vi "buildTestScenario.vi"(0 "TestScenarioFactory in":refnum<class "TestScenarioFactory.lvclass">, 5 "Log":refnum<class "ITestLog.lvclass">, 7 "Test Scenario":T1, 11 "error in (no error)":errorcluster) -> (4 "TestScenarioFactory out":refnum<class "TestScenarioFactory.lvclass">, 6 "ITestScenario.lvclass":refnum<class "ITestScenario.lvclass">, 15 "error out":errorcluster)   [LabVIEW 2015, in "TestScenarioFactory.lvclass"]
uses:
  TestScenarioFactory.lvclass
  Typedefs/TestScenarioTypes.ctl
  TestScenario/ITestScenario/ITestScenario.lvclass
  TestLog/ITestLog/ITestLog.lvclass
  TestScenario/Not Implemented Test/NotImplementedTest.lvclass
  TestScenario/Constant Analog Output Voltage Test/Constant Analog Output Voltage Test.lvclass
  TestScenarioFactory.lvclass/TestScenarioFactory.ctl
  TestScenario/SSR_TTL Low Test/SSR_TTL Low Test.lvclass
  TestScenario/SSR_TTL High Test/SSR_TTL High Test.lvclass
  TestScenario/SM_CW Low Test/SM_CW Low Test.lvclass
  TestScenario/SM_CW High Test/SM_CW High Test.lvclass
  TestScenario/SM_CCW Low Test/SM_CCW Low Test.lvclass
  TestScenario/SM_CCW High Test/SM_CCW High Test.lvclass
  TestScenario/RS232-TXD Low Test/RS232-TXD Low Test.lvclass
  TestScenario/RS232-TXD High Test/RS232-TXD High Test.lvclass
  TestScenario/RS232-RTS Low Test/RS232-RTS Low Test.lvclass
  TestScenario/RS232-RTS High Test/RS232-RTS High Test.lvclass
  TestScenario/RS232-RXD Low Test/RS232-RXD Low Test.lvclass
  TestScenario/RS232-RXD High Test/RS232-RXD High Test.lvclass
  TestScenario/RS232-CTS low Test/RS232-CTS low Test.lvclass
  TestScenario/RS232-CTS High Test/RS232-CTS High Test.lvclass
  TestScenario/Modulated Analog Output Voltage Test/Modulated Analog Output Voltage Test.lvclass
  ConfigureILCStrategy/ConfigureILCROTStrategy/ConfigureILCROTStrategy.lvclass
  ConverterStrategy/ConvertROTRawToEngStrategy/ConvertROTRawToEngStrategy.lvclass
  ConfigureILCStrategy/ConfigureILCDAC1Strategy/ConfigureILCDAC1Strategy.lvclass
  ConverterStrategy/ConvertDACRawToEngStrategy/ConvertDACRawToEngStrategy.lvclass
  Typedefs/ILCBTTypedefs.lvlib
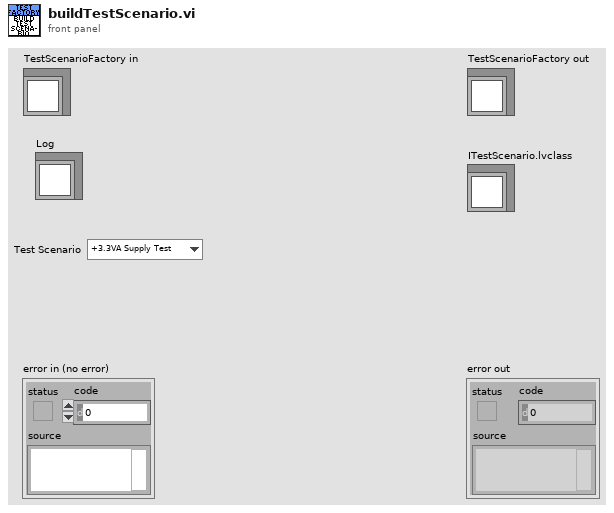
[diagram p1: front panel]
types:
  T1 = typedef "ILCBTTypedefs.lvlib/TestScenarioTypes.ctl" = enum16{"+3.3VA Supply Test", "+3.3VD Supply Test", "+5VA Supply Test", "+5VD Supply Test", "Unique ID Test", "TEDS Status Test", "LIMSW1_TTL Low Test", "LIMSW1_TTL High Test", "LIMSW2_TTL Low Test", "LIMSW2_TTL High Test", "Tachometer Test", "SSR_TTL Low Test", "SSR_TTL High Test", "SM_CW Low Test", "SM_CW High Test", "SM_CCW Low Test", "SM_CCW High Test", "SM_GPI Low Test", "SM_GPI High Test", "CW Motion Without Limit Test", "CW Motion With Limit Test", "CW Motion With Limit Interruption Test", "CW Motion on CCW Limit Test", "CCW Motion Without Limit Test", "CCW Motion With Limit Test", "CCW Motion With Limit Interruption Test", "CCW Motion on CW Limit Test", "RS232-TXD Low Test", "RS232-TXD High Test", "RS232-RTS Low Test", "RS232-RTS High Test", "RS232-RXD Low Test", "RS232-RXD High Test", "RS232-CTS Low Test", "RS232-CTS High Test", "Out_SS Low Test", "Out_SS High Test", "Out_SDI Low Test", "Out_SDI High Test", "Out_SCLK Low Test", "Out_SCLK High Test", "Reset Low Test", "Reset High Test", "1 Channel ADC Test", "3 Channel ADC Test", "5 Channel ADC Test", "Vref Test", "ROT Test", "DAC1 Test", "DAC2 Test", "DAC3 Test", "DAC4 Test", "BIAS Test", "EXC1 Test", "EXC2 Test", "EXC3 Test", "EXC4 Test"}
  T2 = typedef "ILCBTTypedefs.lvlib/ILC Digital Output Test.ctl" = cluster{"DAQ Channel to Read":refnum<k21>, "High Level Value to Test":T3, "High Level Value to Expect":T3, "Low Level Value to Test":T3, "Low Level Value to Expect":T3}
  T3 = typedef "ILCBTTypedefs.lvlib/Digital Signal Level.ctl" = enum16{"Low", "High"}
  T4 = typedef "ILCBTTypedefs.lvlib/MUX Settings.ctl" = cluster{"MUX_AO":T3, "MUX_A1":T3, "MUX_A0 DAQ Channel to Write":refnum<k21>, "MUX_A1 DAQ Channel to Write":refnum<k21>}
  T5 = typedef "ILCBTTypedefs.lvlib/Test Values.ctl" = cluster{"Start Value":dbl, "Stop Value":dbl, "Number of Steps":u16}
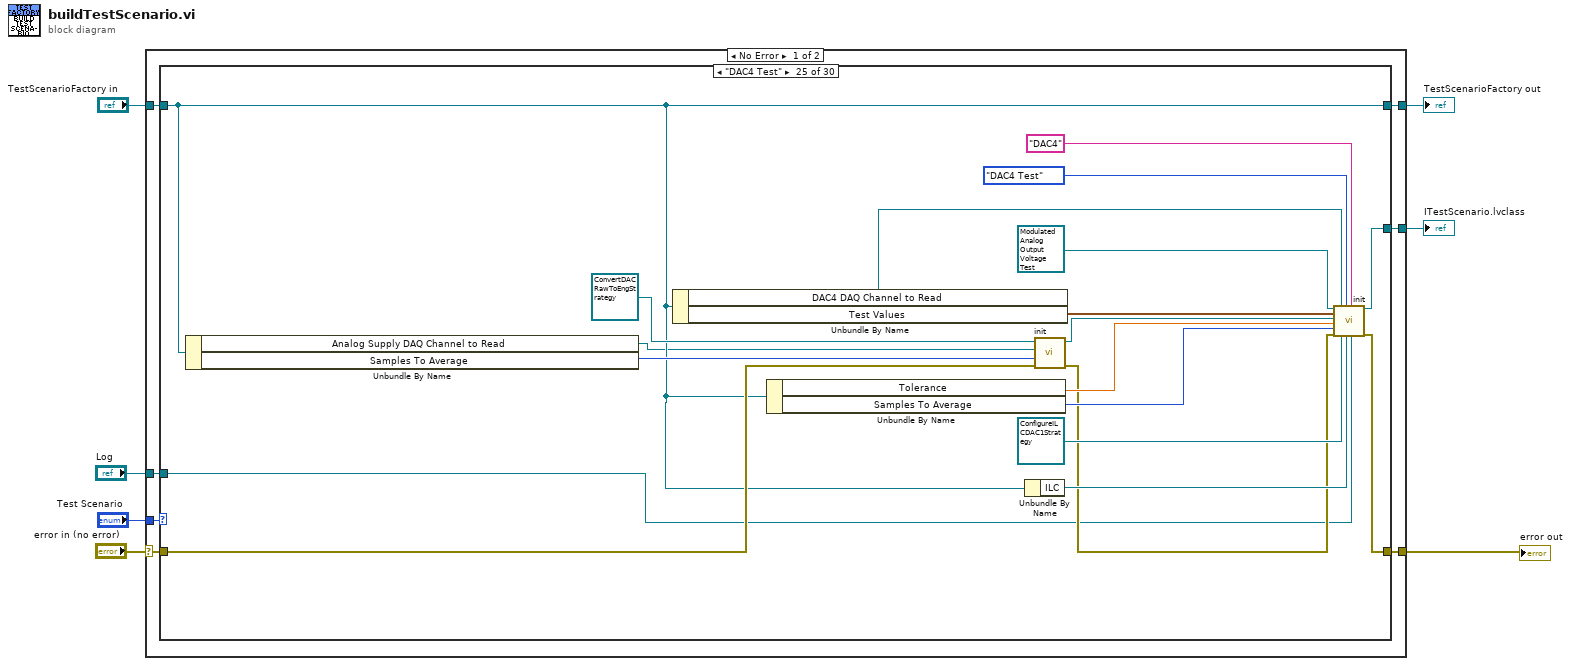
[diagram p0: block diagram]
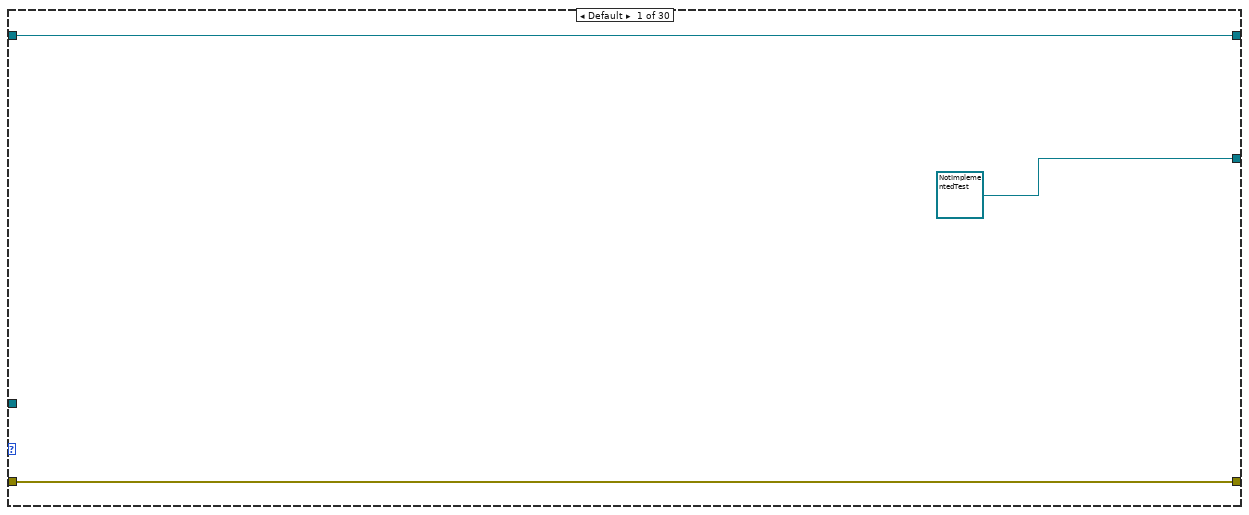
[diagram p2: hidden frame]
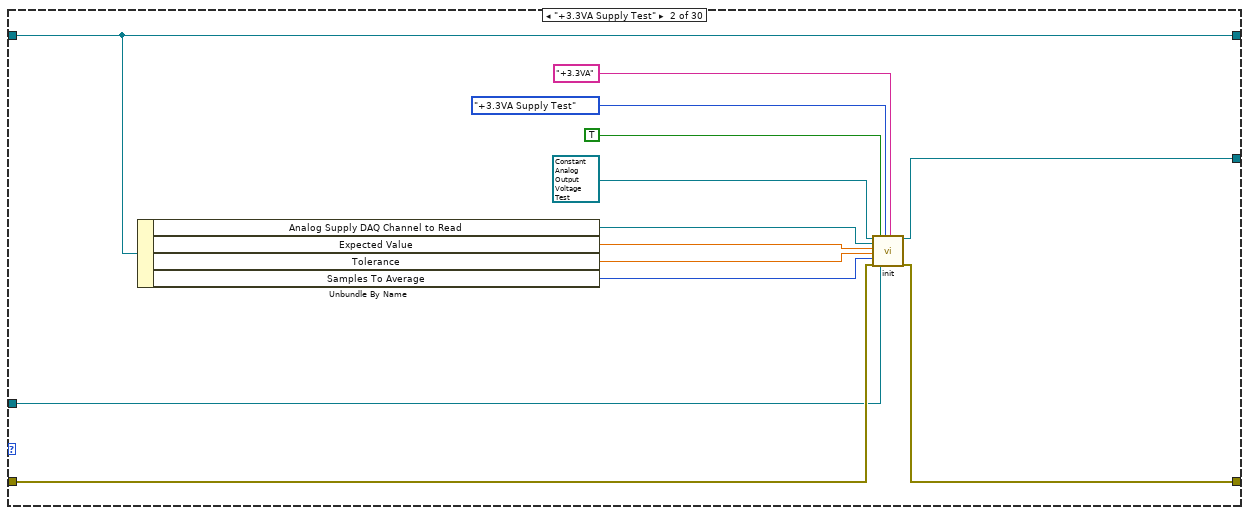
[diagram p3: hidden frame]
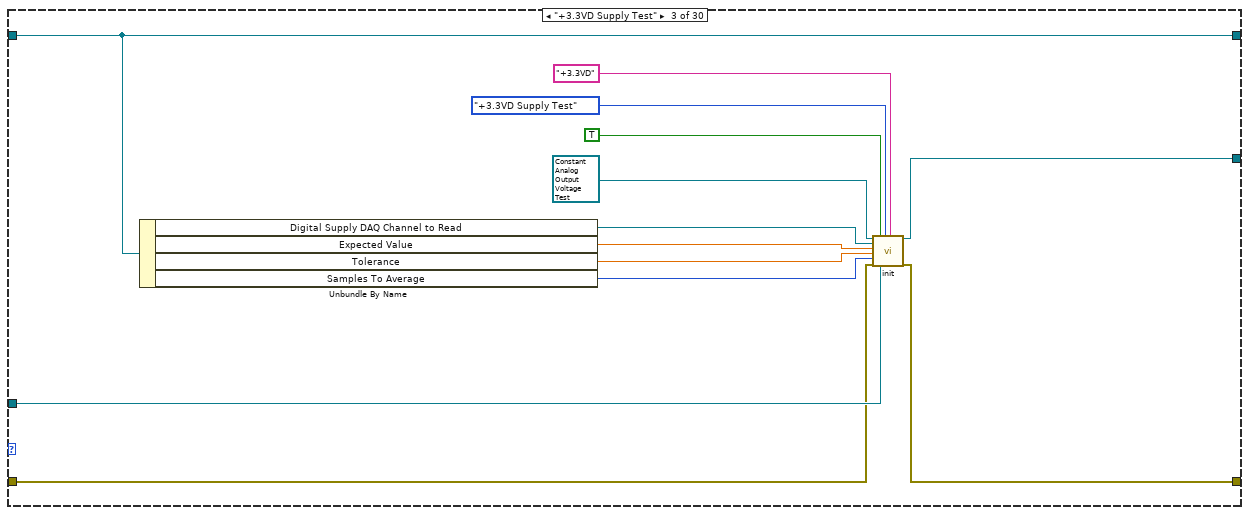
[diagram p4: hidden frame]
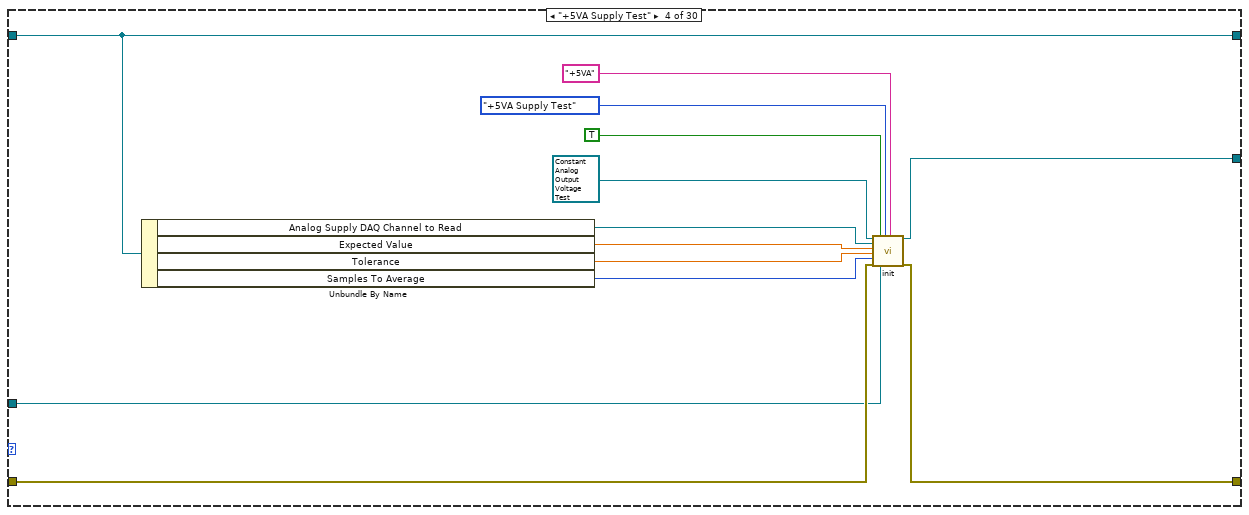
[diagram p5: hidden frame]
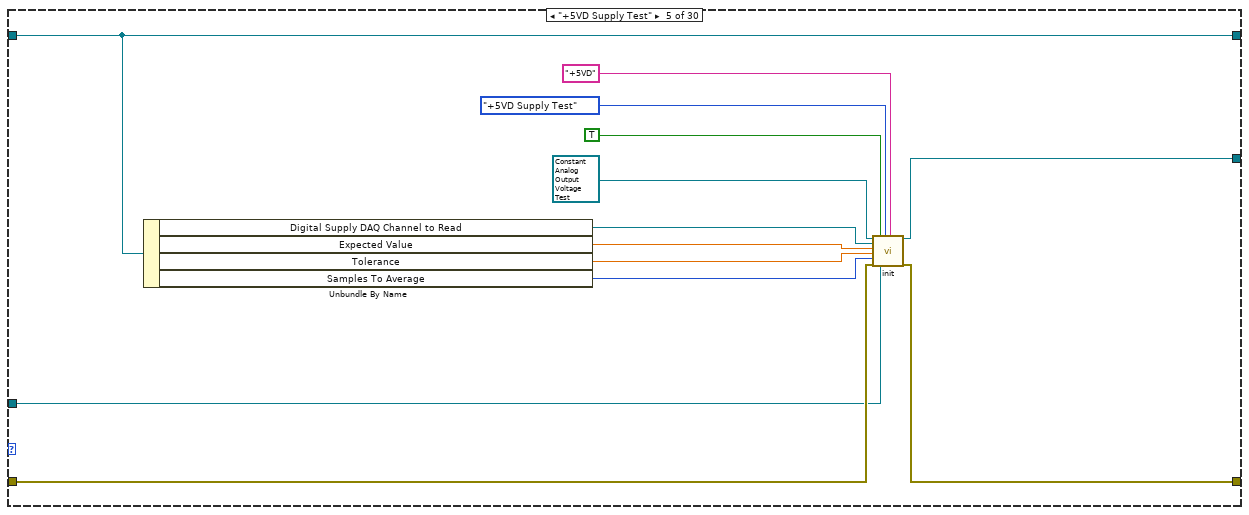
[diagram p6: hidden frame]
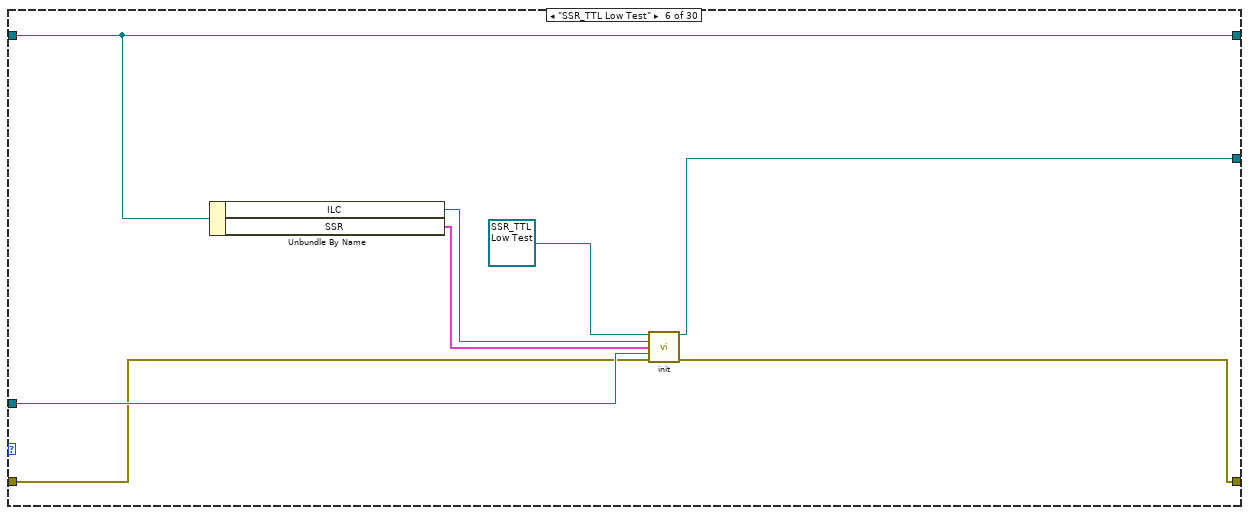
[diagram p7: hidden frame]
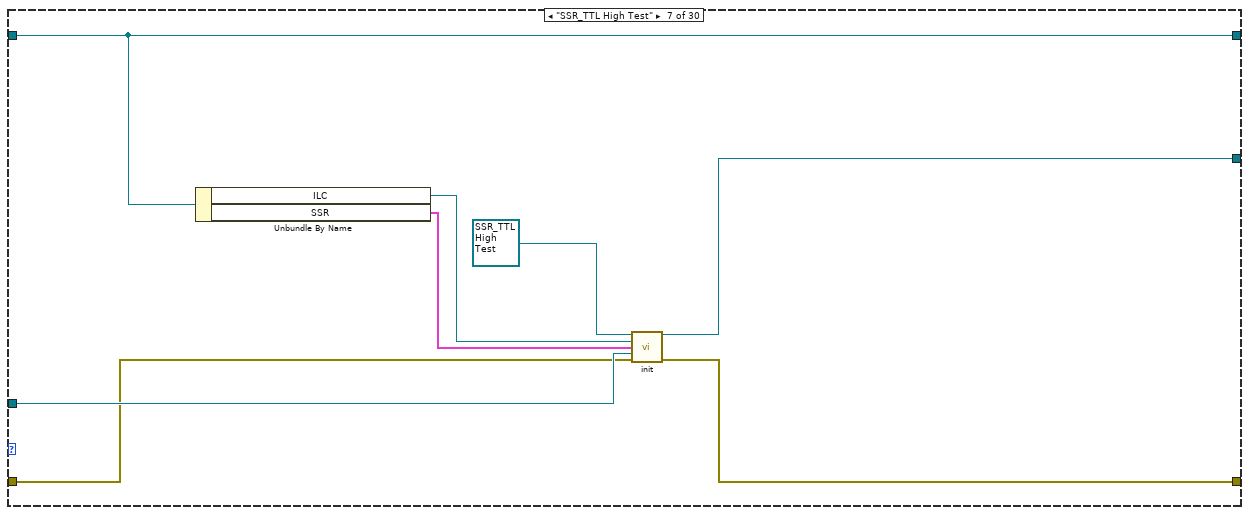
[diagram p8: hidden frame]
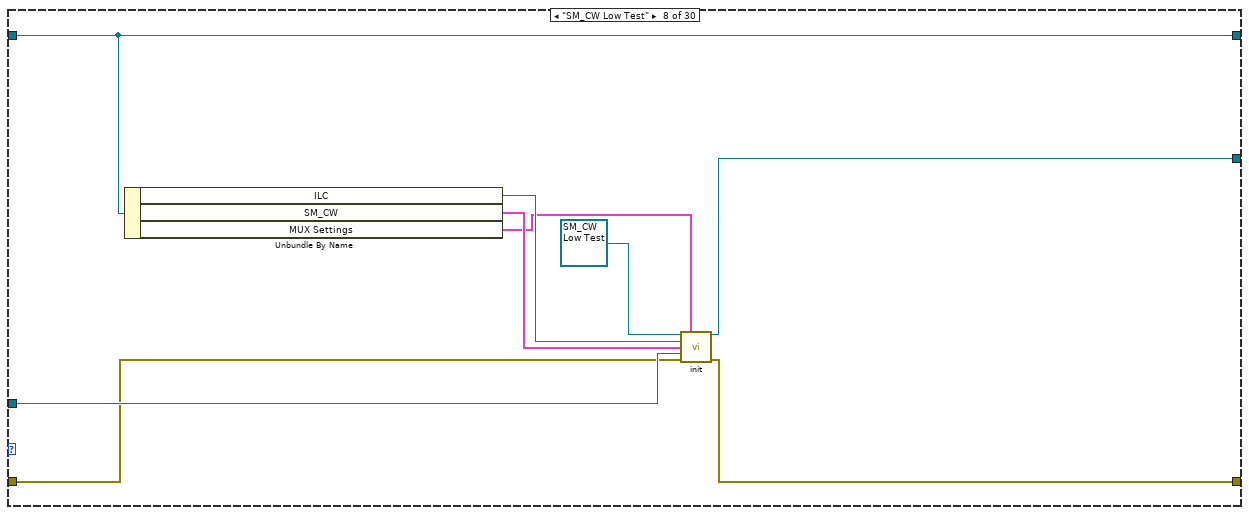
[diagram p9: hidden frame]
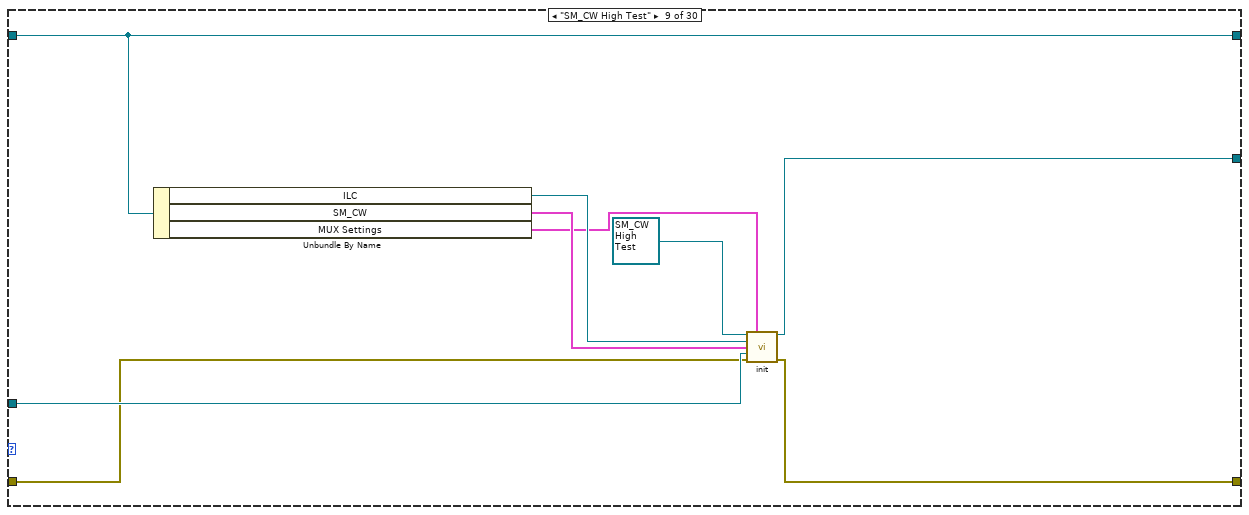
[diagram p10: hidden frame]
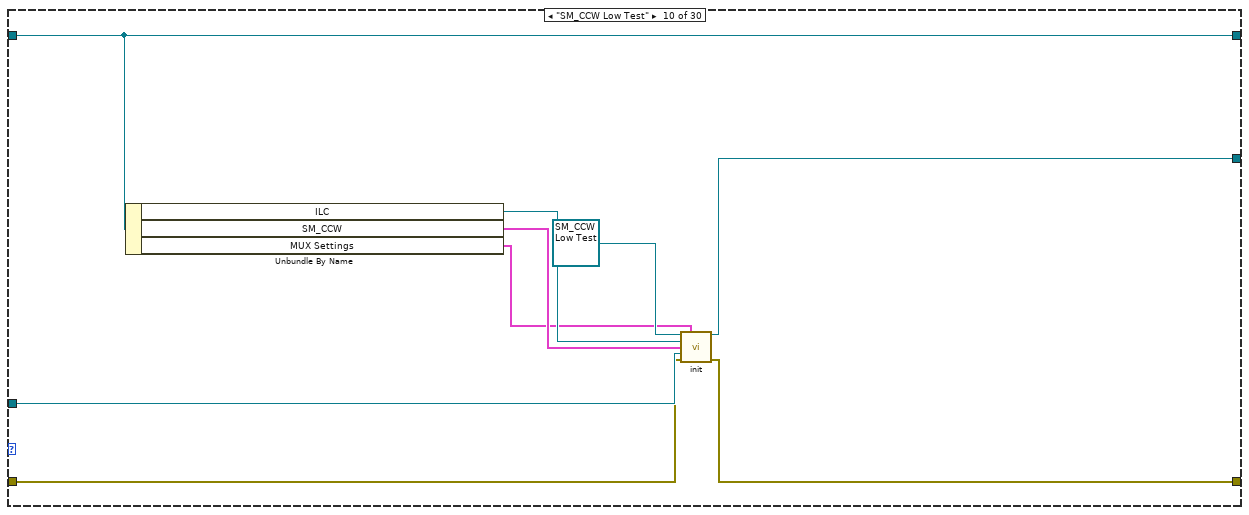
[diagram p11: hidden frame]
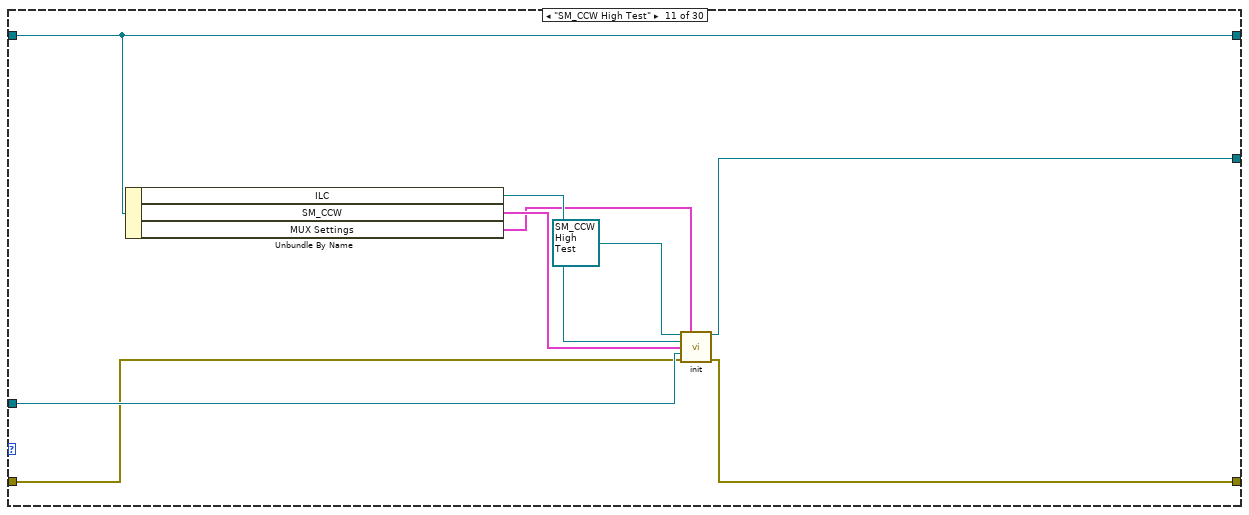
[diagram p12: hidden frame]
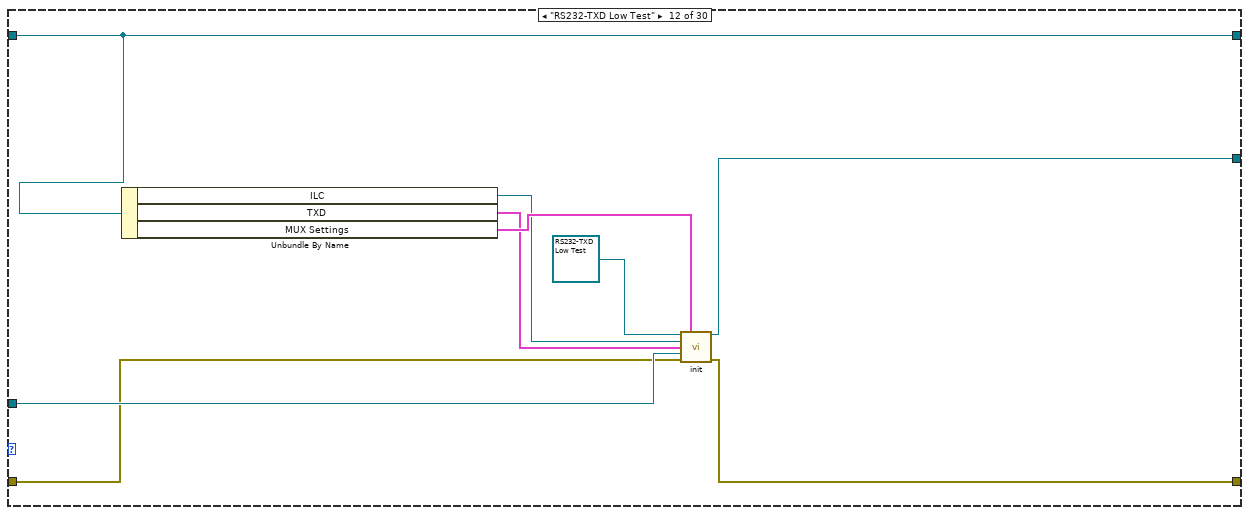
[diagram p13: hidden frame]
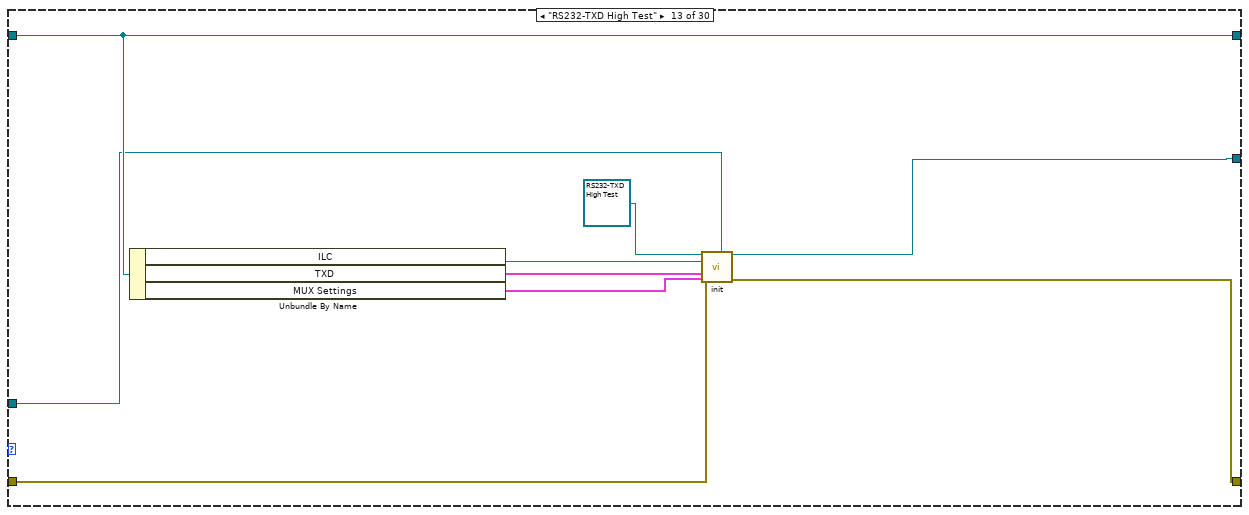
[diagram p14: hidden frame]
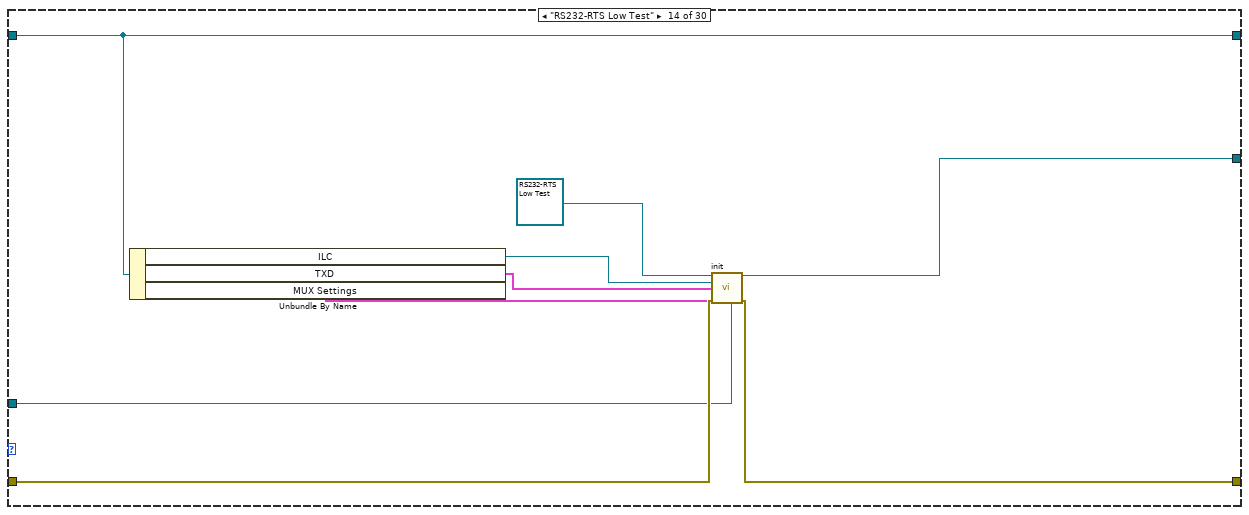
[diagram p15: hidden frame]
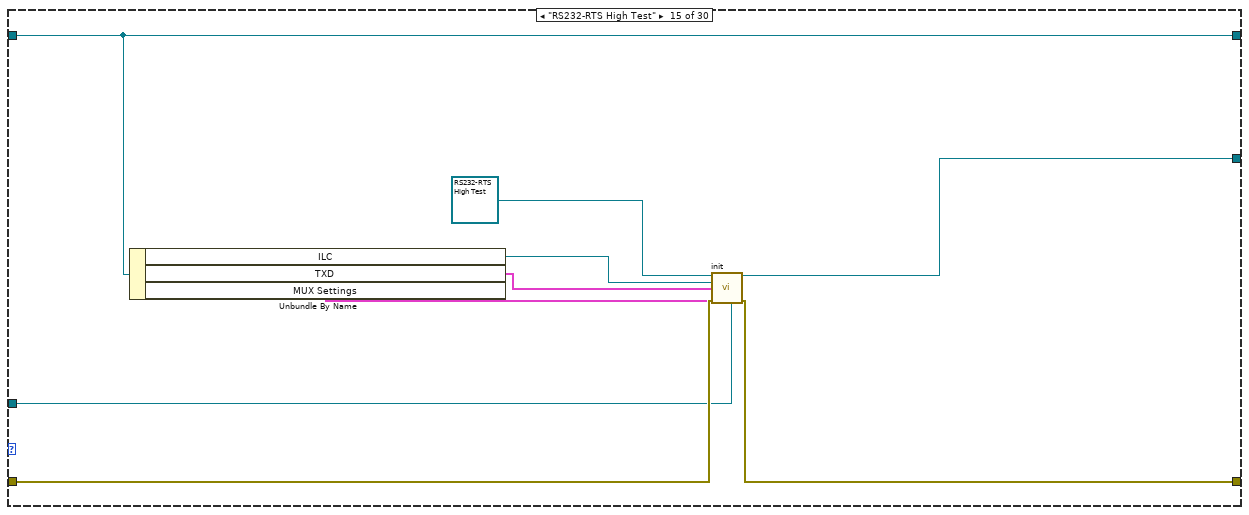
[diagram p16: hidden frame]
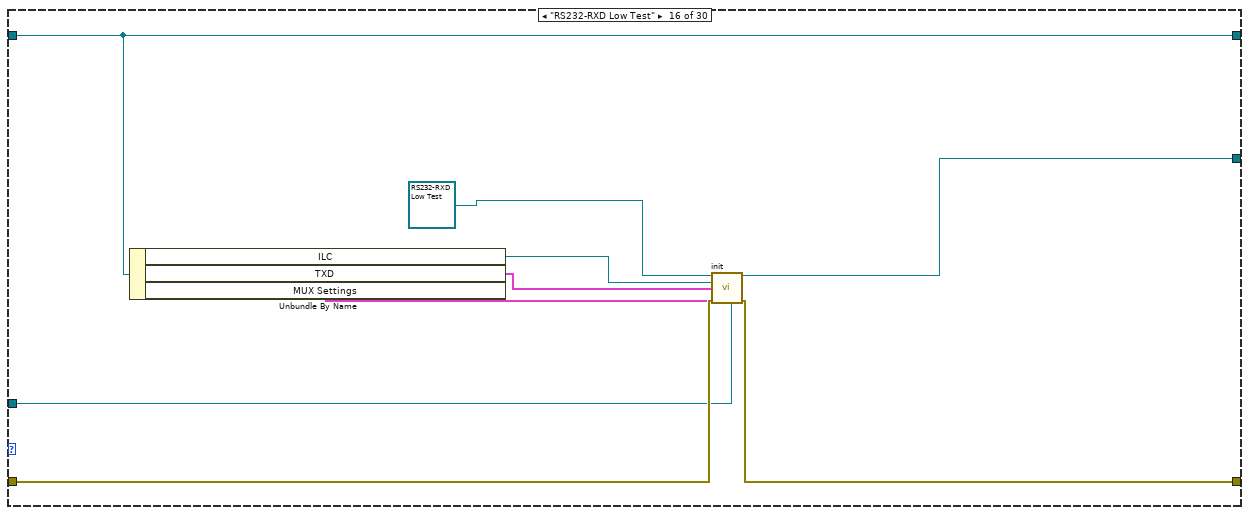
[diagram p17: hidden frame]
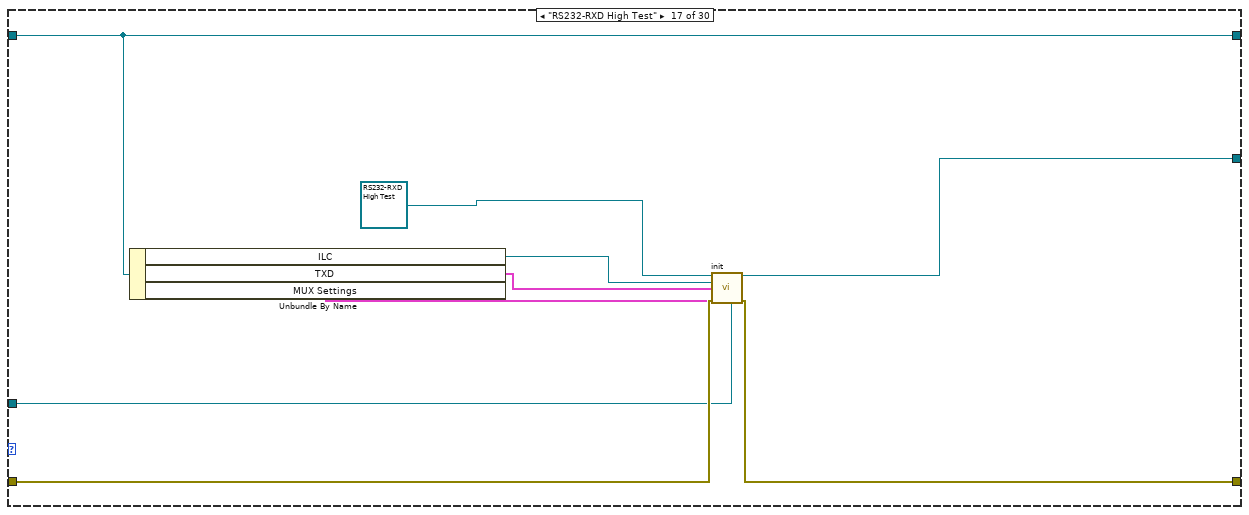
[diagram p18: hidden frame]
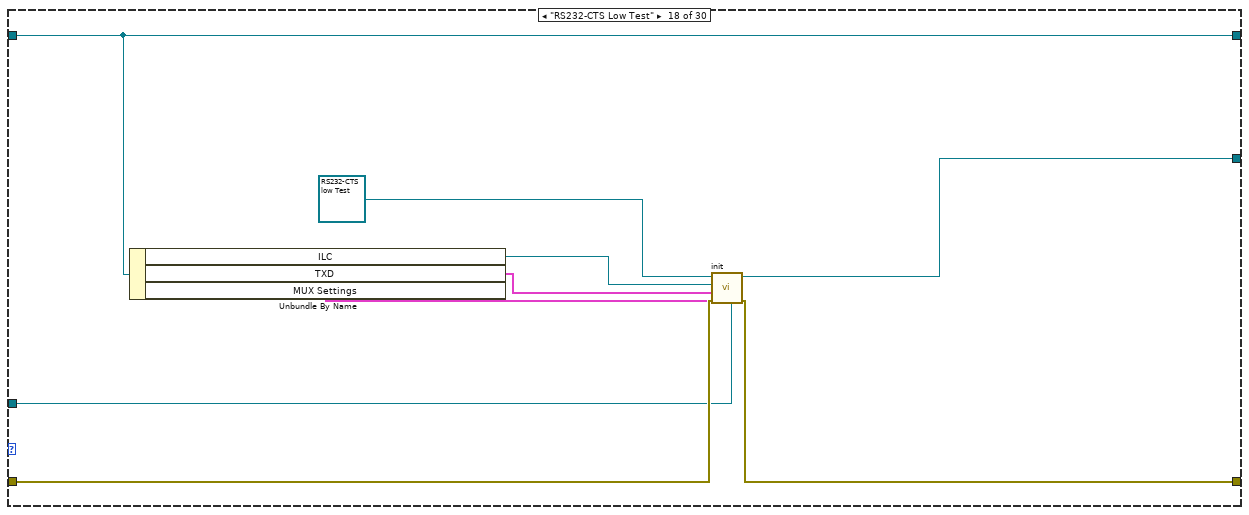
[diagram p19: hidden frame]
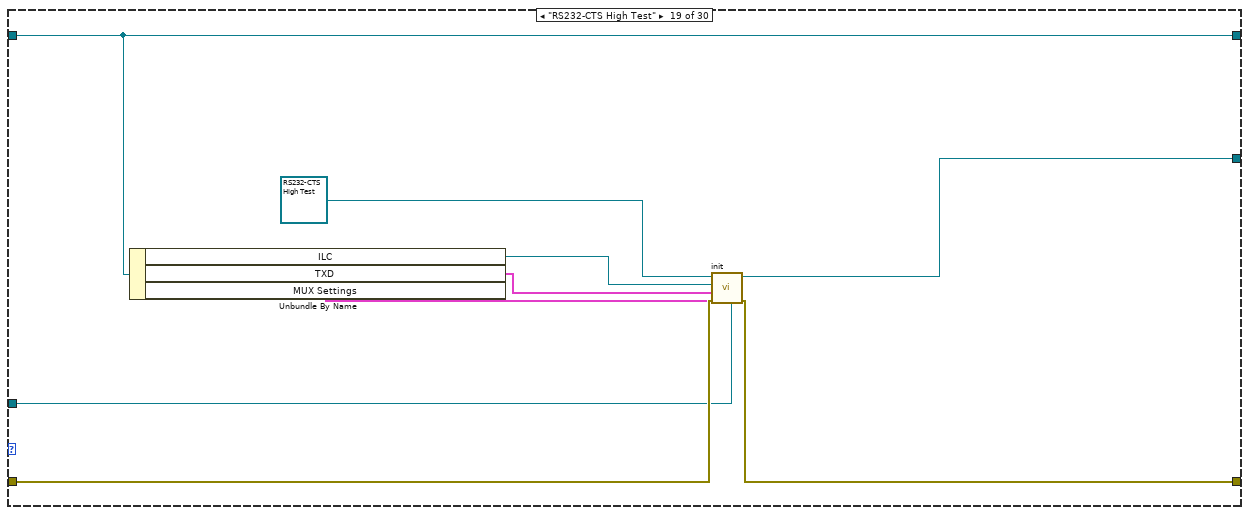
[diagram p20: hidden frame]
diagram:
  n1 = case shown="No Error" "error in (no error)" {
    selector: "error in (no error)" -> [w12 w369]
    tunnel: "Test Scenario" -> [w14 _]
    tunnel: "TestScenarioFactory in" -> [w13 w368]
    tunnel: [w11 w369] -> w2
    tunnel: [w8 w368] -> w5
    tunnel: "Log" -> [w9 _]
    tunnel: [w10 refnum<class "ITestScenario.lvclass"> refnum ("ITestScenario.lvclass")] -> w4
    frame No Error {
      n2 = case shown="\"DAC4 Test\"" w14 {
        tunnel: w13 -> [w17 w30 w33 w48 w57 w73 w81 w90 w99 w108 w117 w122 w139 w148 w157 w166 w175 w184 w193 w194 w213 w227 w246 w265 w284 w302 w319 w330 w341 w354]
        tunnel: w12 -> [w16 w27 w34 w45 w60 w72 w78 w87 w96 w105 w114 w125 w133 w147 w156 w165 w174 w183 w192 w197 w207 w229 w248 w267 w286 w305 w317 w332 w344 w357]
        tunnel: [w16 w18 w31 w46 w61 w75 w83 w91 w100 w111 w120 w124 w132 w146 w155 w164 w173 w182 w191 w196 w222 w231 w250 w269 w288 w304 w316 w328 w343 w356] -> w11
        tunnel: [refnum<class "NotImplementedTest.lvclass"> refnum ("NotImplementedTest.lvclass") w28 w32 w47 w58 w74 w82 w92 w101 w109 w119 w123 w137 w140 w150 w159 w168 w177 w186 w195 w221 w230 w249 w268 w287 w303 w315 w329 w342 w355] -> w10
        tunnel: w9 -> [_ w26 w35 w44 w59 w76 w84 w93 w102 w110 w118 w126 w135 w144 w154 w163 w172 w181 w190 w198 w215 w228 w247 w266 w285 w306 w318 w331 w345 w358]
        tunnel: [w17 w30 w33 w48 w57 w73 w81 w90 w99 w108 w117 w122 w139 w148 w157 w166 w175 w184 w193 w194 w213 w227 w246 w265 w284 w302 w319 w330 w341 w354] -> w8
        frame Default {
        }
        frame "+3.3VA Supply Test" {
          n3 = Unbundle By Name(w30) -> ("Analog Supply DAQ Channel to Read"=w22:refnum<k21>, "Expected Value"=w23:dbl, "Tolerance"=w24:dbl, "Samples To Average"=w25:i32)
          n4 = call "init.vi"("Constant Analog Output Voltage Test in"=refnum<class "Constant Analog Output Voltage Test.lvclass"> refnum ("Constant Analog Input Voltage Test.lvclass"), "DAQ Channel"=w22, "Expected Value"=w23, "Tolerance"=w24, "Samples To Average"=w25, "error in (no error)"=w27, "MustPass?"=TRUE, "Log"=w26, "Test Scenario"=TestScenarioTypes."+3.3VA Supply Test", "Signal Name"="+3.3VA") -> ("Constant Analog Output Voltage Test  out"=w28:refnum<class "Constant Analog Output Voltage Test.lvclass">, "error out"=w18:errorcluster)  [unwired: 8 in]
        }
        frame "+3.3VD Supply Test" {
          n5 = Unbundle By Name(w33) -> ("Digital Supply DAQ Channel to Read"=w39:refnum<k21>, "Expected Value"=w40:dbl, "Tolerance"=w41:dbl, "Samples To Average"=w42:i32)
          n6 = call "init.vi"("Constant Analog Output Voltage Test in"=refnum<class "Constant Analog Output Voltage Test.lvclass"> refnum ("Constant Analog Input Voltage Test.lvclass"), "DAQ Channel"=w39, "Expected Value"=w40, "Tolerance"=w41, "Samples To Average"=w42, "error in (no error)"=w34, "MustPass?"=TRUE, "Log"=w35, "Test Scenario"=TestScenarioTypes."+3.3VD Supply Test", "Signal Name"="+3.3VD") -> ("Constant Analog Output Voltage Test  out"=w32:refnum<class "Constant Analog Output Voltage Test.lvclass">, "error out"=w31:errorcluster)  [unwired: 8 in]
        }
        frame "+5VA Supply Test" {
          n7 = Unbundle By Name(w48) -> ("Analog Supply DAQ Channel to Read"=w52:refnum<k21>, "Expected Value"=w53:dbl, "Tolerance"=w54:dbl, "Samples To Average"=w55:i32)
          n8 = call "init.vi"("Constant Analog Output Voltage Test in"=refnum<class "Constant Analog Output Voltage Test.lvclass"> refnum ("Constant Analog Input Voltage Test.lvclass"), "DAQ Channel"=w52, "Expected Value"=w53, "Tolerance"=w54, "Samples To Average"=w55, "error in (no error)"=w45, "MustPass?"=TRUE, "Log"=w44, "Test Scenario"=TestScenarioTypes."+5VA Supply Test", "Signal Name"="+5VA") -> ("Constant Analog Output Voltage Test  out"=w47:refnum<class "Constant Analog Output Voltage Test.lvclass">, "error out"=w46:errorcluster)  [unwired: 8 in]
        }
        frame "+5VD Supply Test" {
          n9 = Unbundle By Name(w57) -> ("Digital Supply DAQ Channel to Read"=w66:refnum<k21>, "Expected Value"=w65:dbl, "Tolerance"=w64:dbl, "Samples To Average"=w63:i32)
          n10 = call "init.vi"("Constant Analog Output Voltage Test in"=refnum<class "Constant Analog Output Voltage Test.lvclass"> refnum ("Constant Analog Input Voltage Test.lvclass"), "DAQ Channel"=w66, "Expected Value"=w65, "Tolerance"=w64, "Samples To Average"=w63, "error in (no error)"=w60, "MustPass?"=TRUE, "Log"=w59, "Test Scenario"=TestScenarioTypes."+5VD Supply Test", "Signal Name"="+5VD") -> ("Constant Analog Output Voltage Test  out"=w58:refnum<class "Constant Analog Output Voltage Test.lvclass">, "error out"=w61:errorcluster)  [unwired: 8 in]
        }
        frame "SSR_TTL Low Test" {
          n11 = Unbundle By Name(w73) -> ("ILC"=w71:refnum<class "ILC.lvclass">, "SSR"=w70:T2)
          n12 = call "init.vi"("SSR_TTL Low Test in"=refnum<class "SSR_TTL Low Test.lvclass"> refnum ("SSR_TTL Low Test.lvclass"), "ILC"=w71, "ILC Digital Output Test"=w70, "Log"=w76, "error in (no error)"=w72) -> ("SSR_TTL Low Test out"=w74:refnum<class "SSR_TTL Low Test.lvclass">, "error out"=w75:errorcluster)  [unwired: 9 in]
        }
        frame "SSR_TTL High Test" {
          n13 = Unbundle By Name(w81) -> ("ILC"=w80:refnum<class "ILC.lvclass">, "SSR"=w79:T2)
          n14 = call "init.vi"("SSR_TTL High Test in"=refnum<class "SSR_TTL High Test.lvclass"> refnum ("SSR_TTL High Test.lvclass"), "ILC"=w80, "ILC Digital Output Test"=w79, "Log"=w84, "error in (no error)"=w78) -> ("SSR_TTL High Test out"=w82:refnum<class "SSR_TTL High Test.lvclass">, "error out"=w83:errorcluster)  [unwired: 9 in]
        }
        frame "SM_CW Low Test" {
          n15 = Unbundle By Name(w90) -> ("ILC"=w89:refnum<class "ILC.lvclass">, "SM_CW"=w88:T2, "MUX Settings"=w86:T4)
          n16 = call "init.vi"("SM_CW Low Test in"=refnum<class "SM_CW Low Test.lvclass"> refnum ("SM_CW Low Test.lvclass"), "MUX Settings"=w86, "ILC"=w89, "ILC Digital Output Test"=w88, "Log"=w93, "error in (no error)"=w87) -> ("SM_CW Low Test out"=w92:refnum<class "SM_CW Low Test.lvclass">, "error out"=w91:errorcluster)  [unwired: 8 in]
        }
        frame "SM_CW High Test" {
          n17 = Unbundle By Name(w99) -> ("ILC"=w97:refnum<class "ILC.lvclass">, "SM_CW"=w98:T2, "MUX Settings"=w95:T4)
          n18 = call "init.vi"("SM_CW High Test in"=refnum<class "SM_CW High Test.lvclass"> refnum ("SM_CW High Test.lvclass"), "MUX Settings"=w95, "ILC"=w97, "ILC Digital Output Test"=w98, "Log"=w102, "error in (no error)"=w96) -> ("SM_CW High Test out"=w101:refnum<class "SM_CW High Test.lvclass">, "error out"=w100:errorcluster)  [unwired: 8 in]
        }
        frame "SM_CCW Low Test" {
          n19 = Unbundle By Name(w108) -> ("ILC"=w107:refnum<class "ILC.lvclass">, "SM_CCW"=w106:T2, "MUX Settings"=w104:T4)
          n20 = call "init.vi"("SM_CCW Low Test in"=refnum<class "SM_CCW Low Test.lvclass"> refnum ("SM_CCW Low Test.lvclass"), "MUX Settings"=w104, "ILC"=w107, "ILC Digital Output Test"=w106, "Log"=w110, "error in (no error)"=w105) -> ("SM_CCW Low Test out"=w109:refnum<class "SM_CCW Low Test.lvclass">, "error out"=w111:errorcluster)  [unwired: 8 in]
        }
        frame "SM_CCW High Test" {
          n21 = Unbundle By Name(w117) -> ("ILC"=w116:refnum<class "ILC.lvclass">, "SM_CCW"=w115:T2, "MUX Settings"=w113:T4)
          n22 = call "init.vi"("SM_CCW High Test in"=refnum<class "SM_CCW High Test.lvclass"> refnum ("SM_CCW High Test.lvclass"), "MUX Settings"=w113, "ILC"=w116, "ILC Digital Output Test"=w115, "Log"=w118, "error in (no error)"=w114) -> ("SM_CCW High Test out"=w119:refnum<class "SM_CCW High Test.lvclass">, "error out"=w120:errorcluster)  [unwired: 8 in]
        }
        frame "RS232-TXD Low Test" {
          n23 = Unbundle By Name(w122) -> ("ILC"=w128:refnum<class "ILC.lvclass">, "TXD"=w127:T2, "MUX Settings"=w130:T4)
          n24 = call "init.vi"("RS232-TXD Low Test in"=refnum<class "RS232-TXD Low Test.lvclass"> refnum ("RS232-TXD Low Test.lvclass"), "MUX Settings"=w130, "ILC"=w128, "ILC Digital Output Test"=w127, "Log"=w126, "error in (no error)"=w125) -> ("RS232-TXD Low Test out"=w123:refnum<class "RS232-TXD Low Test.lvclass">, "error out"=w124:errorcluster)  [unwired: 8 in]
        }
        frame "RS232-TXD High Test" {
          n25 = Unbundle By Name(w139) -> ("ILC"=w136:refnum<class "ILC.lvclass">, "TXD"=w134:T2, "MUX Settings"=w131:T4)
          n26 = call "init.vi"("RS232-TXD High Test in"=refnum<class "RS232-TXD High Test.lvclass"> refnum ("RS232-TXD High Test.lvclass"), "MUX Settings"=w131, "ILC"=w136, "ILC Digital Output Test"=w134, "Log"=w135, "error in (no error)"=w133) -> ("RS232-TXD High Test out"=w137:refnum<class "RS232-TXD High Test.lvclass">, "error out"=w132:errorcluster)  [unwired: 8 in]
        }
        frame "RS232-RTS Low Test" {
          n27 = Unbundle By Name(w148) -> ("ILC"=w143:refnum<class "ILC.lvclass">, "TXD"=w142:T2, "MUX Settings"=w141:T4)
          n28 = call "init.vi"("RS232-RTS Low Test in"=refnum<class "RS232-RTS Low Test.lvclass"> refnum ("RS232-RTS Low Test.lvclass"), "MUX Settings"=w141, "ILC"=w143, "ILC Digital Output Test"=w142, "Log"=w144, "error in (no error)"=w147) -> ("RS232-RTS Low Test out"=w140:refnum<class "RS232-RTS Low Test.lvclass">, "error out"=w146:errorcluster)  [unwired: 8 in]
        }
        frame "RS232-RTS High Test" {
          n29 = Unbundle By Name(w157) -> ("ILC"=w153:refnum<class "ILC.lvclass">, "TXD"=w152:T2, "MUX Settings"=w151:T4)
          n30 = call "init.vi"("RS232-RTS High Test in"=refnum<class "RS232-RTS High Test.lvclass"> refnum ("RS232-RTS High Test.lvclass"), "MUX Settings"=w151, "ILC"=w153, "ILC Digital Output Test"=w152, "Log"=w154, "error in (no error)"=w156) -> ("RS232-RTS High Test out"=w150:refnum<class "RS232-RTS High Test.lvclass">, "error out"=w155:errorcluster)  [unwired: 8 in]
        }
        frame "RS232-RXD Low Test" {
          n31 = Unbundle By Name(w166) -> ("ILC"=w162:refnum<class "ILC.lvclass">, "TXD"=w161:T2, "MUX Settings"=w160:T4)
          n32 = call "init.vi"("RS232-RXD Low Test in"=refnum<class "RS232-RXD Low Test.lvclass"> refnum ("RS232-RXD Low Test.lvclass"), "MUX Settings"=w160, "ILC"=w162, "ILC Digital Output Test"=w161, "Log"=w163, "error in (no error)"=w165) -> ("RS232-RXD Low Test out"=w159:refnum<class "RS232-RXD Low Test.lvclass">, "error out"=w164:errorcluster)  [unwired: 8 in]
        }
        frame "RS232-RXD High Test" {
          n33 = Unbundle By Name(w175) -> ("ILC"=w171:refnum<class "ILC.lvclass">, "TXD"=w170:T2, "MUX Settings"=w169:T4)
          n34 = call "init.vi"("RS232-RXD High Test in"=refnum<class "RS232-RXD High Test.lvclass"> refnum ("RS232-RXD High Test.lvclass"), "MUX Settings"=w169, "ILC"=w171, "ILC Digital Output Test"=w170, "Log"=w172, "error in (no error)"=w174) -> ("RS232-RXD High Test out"=w168:refnum<class "RS232-RXD High Test.lvclass">, "error out"=w173:errorcluster)  [unwired: 8 in]
        }
        frame "RS232-CTS Low Test" {
          n35 = Unbundle By Name(w184) -> ("ILC"=w180:refnum<class "ILC.lvclass">, "TXD"=w179:T2, "MUX Settings"=w178:T4)
          n36 = call "init.vi"("MUX Settings"=w178, "Log"=w181, "error in (no error)"=w183, "ILC Digital Output Test"=w179, "ILC"=w180, "RS232-CTS Low Test in"=refnum<class "RS232-CTS low Test.lvclass"> refnum ("RS232-CTS low Test.lvclass")) -> ("error out"=w182:errorcluster, "RS232-CTS Low Test out"=w177:refnum<class "RS232-CTS low Test.lvclass">)  [unwired: 4 in]
        }
        frame "RS232-CTS High Test" {
          n37 = Unbundle By Name(w193) -> ("ILC"=w189:refnum<class "ILC.lvclass">, "TXD"=w188:T2, "MUX Settings"=w187:T4)
          n38 = call "init.vi"("MUX Settings"=w187, "Log"=w190, "error in (no error)"=w192, "ILC Digital Output Test"=w188, "ILC"=w189, "RS232-CTS High Test in"=refnum<class "RS232-CTS High Test.lvclass"> refnum ("RS232-CTS High Test.lvclass")) -> ("error out"=w191:errorcluster, "RS232-CTS High Test out"=w186:refnum<class "RS232-CTS High Test.lvclass">)  [unwired: 4 in]
        }
        frame "Vref Test" {
          n39 = Unbundle By Name(w194) -> ("DAQ Channel to Read"=w202:refnum<k21>, "Expected Value"=w203:dbl, "Tolerance"=w204:dbl, "Samples To Average"=w205:i32)
          n40 = call "init.vi"("Constant Analog Output Voltage Test in"=refnum<class "Constant Analog Output Voltage Test.lvclass"> refnum ("Constant Analog Input Voltage Test.lvclass"), "DAQ Channel"=w202, "Expected Value"=w203, "Tolerance"=w204, "Samples To Average"=w205, "error in (no error)"=w197, "MustPass?"=FALSE, "Log"=w198, "Test Scenario"=TestScenarioTypes."Vref Test", "Signal Name"="Vref") -> ("Constant Analog Output Voltage Test  out"=w195:refnum<class "Constant Analog Output Voltage Test.lvclass">, "error out"=w196:errorcluster)  [unwired: 8 in]
        }
        frame "ROT Test" {
          n41 = Unbundle By Name(w213) -> ("DAQ Channel to Read"=w211:refnum<k21>, "Samples To Average"=w210:i32)
          n42 = Unbundle By Name(w213) -> ("DAQ Channel to Read"=w220:refnum<k21>, "Test Values"=w219:T5)
          n43 = Unbundle By Name(w213) -> ("Tolerance"=w217:dbl, "Samples To Average"=w216:i32)
          n44 = Unbundle By Name(w213) -> ("ILC"=w214:refnum<class "ILC.lvclass">)
          n45 = call "init.vi"("error in (no error)"=w207, "Samples To Average"=w210, "Vref Channel"=w211, "ConvertROTRawToEngStrategy in"=refnum<class "ConvertROTRawToEngStrategy.lvclass"> refnum ("ConvertROTRawToEngStrategy.lvclass")) -> ("error out"=w208:errorcluster, "ConvertROTRawToEngStrategy out"=w209:refnum<class "ConvertROTRawToEngStrategy.lvclass">)  [unwired: 6 in]
          n46 = call "init.vi"("Constant Analog Output Voltage Test in"=refnum<class "Modulated Analog Output Voltage Test.lvclass"> refnum ("Constant Analog Input Voltage Test.lvclass"), "Test Values"=w219, "ConvertStrategy"=w209, "Tolerance"=w217, "Samples To Average"=w216, "error in (no error)"=w208, "DAQ Channel"=w220, "ConfigureILCStrategy"=refnum<class "ConfigureILCROTStrategy.lvclass"> refnum ("ConfigureILCROTStrategy.lvclass"), "Test Scenario"=TestScenarioTypes."ROT Test", "ILC"=w214, "Signal Name"="ROT", "Log"=w215) -> ("Constant Analog Output Voltage Test  out"=w221:refnum<class "Modulated Analog Output Voltage Test.lvclass">, "error out"=w222:errorcluster)  [unwired: 6 in]
        }
        frame "DAC1 Test" {
          n47 = Unbundle By Name(w227) -> ("Analog Supply DAQ Channel to Read"=w226:refnum<k21>, "Samples To Average"=w234:i32)
          n48 = Unbundle By Name(w227) -> ("DAC1 DAQ Channel to Read"=w241:refnum<k21>, "Test Values"=w240:T5)
          n49 = Unbundle By Name(w227) -> ("Tolerance"=w238:dbl, "Samples To Average"=w237:i32)
          n50 = Unbundle By Name(w227) -> ("ILC"=w236:refnum<class "ILC.lvclass">)
          n51 = call "init.vi"("error in (no error)"=w229, "Samples To Average"=w234, "+5VA Channel"=w226, "ConvertDACRawToEngStrategy in"=refnum<class "ConvertDACRawToEngStrategy.lvclass"> refnum ("ConvertDACRawToEngStrategy.lvclass")) -> ("error out"=w232:errorcluster, "ConvertDACRawToEngStrategy out"=w233:refnum<class "ConvertDACRawToEngStrategy.lvclass">)  [unwired: 6 in]
          n52 = call "init.vi"("Constant Analog Output Voltage Test in"=refnum<class "Modulated Analog Output Voltage Test.lvclass"> refnum ("Constant Analog Input Voltage Test.lvclass"), "Test Values"=w240, "ConvertStrategy"=w233, "Tolerance"=w238, "Samples To Average"=w237, "error in (no error)"=w232, "DAQ Channel"=w241, "ConfigureILCStrategy"=refnum<class "ConfigureILCDAC1Strategy.lvclass"> refnum ("ConfigureILCDAC1Strategy.lvclass"), "Test Scenario"=TestScenarioTypes."DAC1 Test", "ILC"=w236, "Signal Name"="DAC1", "Log"=w228) -> ("Constant Analog Output Voltage Test  out"=w230:refnum<class "Modulated Analog Output Voltage Test.lvclass">, "error out"=w231:errorcluster)  [unwired: 6 in]
        }
        frame "DAC2 Test" {
          n53 = Unbundle By Name(w246) -> ("Analog Supply DAQ Channel to Read"=w245:refnum<k21>, "Samples To Average"=w253:i32)
          n54 = Unbundle By Name(w246) -> ("DAC2 DAQ Channel to Read"=w260:refnum<k21>, "Test Values"=w259:T5)
          n55 = Unbundle By Name(w246) -> ("Tolerance"=w257:dbl, "Samples To Average"=w256:i32)
          n56 = Unbundle By Name(w246) -> ("ILC"=w255:refnum<class "ILC.lvclass">)
          n57 = call "init.vi"("error in (no error)"=w248, "Samples To Average"=w253, "+5VA Channel"=w245, "ConvertDACRawToEngStrategy in"=refnum<class "ConvertDACRawToEngStrategy.lvclass"> refnum ("ConvertDACRawToEngStrategy.lvclass")) -> ("error out"=w251:errorcluster, "ConvertDACRawToEngStrategy out"=w252:refnum<class "ConvertDACRawToEngStrategy.lvclass">)  [unwired: 6 in]
          n58 = call "init.vi"("Constant Analog Output Voltage Test in"=refnum<class "Modulated Analog Output Voltage Test.lvclass"> refnum ("Constant Analog Input Voltage Test.lvclass"), "Test Values"=w259, "ConvertStrategy"=w252, "Tolerance"=w257, "Samples To Average"=w256, "error in (no error)"=w251, "DAQ Channel"=w260, "ConfigureILCStrategy"=refnum<class "ConfigureILCDAC1Strategy.lvclass"> refnum ("ConfigureILCDAC1Strategy.lvclass"), "Test Scenario"=TestScenarioTypes."DAC2 Test", "ILC"=w255, "Signal Name"="DAC2", "Log"=w247) -> ("Constant Analog Output Voltage Test  out"=w249:refnum<class "Modulated Analog Output Voltage Test.lvclass">, "error out"=w250:errorcluster)  [unwired: 6 in]
        }
        frame "DAC3 Test" {
          n59 = Unbundle By Name(w265) -> ("Analog Supply DAQ Channel to Read"=w264:refnum<k21>, "Samples To Average"=w272:i32)
          n60 = Unbundle By Name(w265) -> ("DAC3 DAQ Channel to Read"=w279:refnum<k21>, "Test Values"=w278:T5)
          n61 = Unbundle By Name(w265) -> ("Tolerance"=w276:dbl, "Samples To Average"=w275:i32)
          n62 = Unbundle By Name(w265) -> ("ILC"=w274:refnum<class "ILC.lvclass">)
          n63 = call "init.vi"("error in (no error)"=w267, "Samples To Average"=w272, "+5VA Channel"=w264, "ConvertDACRawToEngStrategy in"=refnum<class "ConvertDACRawToEngStrategy.lvclass"> refnum ("ConvertDACRawToEngStrategy.lvclass")) -> ("error out"=w270:errorcluster, "ConvertDACRawToEngStrategy out"=w271:refnum<class "ConvertDACRawToEngStrategy.lvclass">)  [unwired: 6 in]
          n64 = call "init.vi"("Constant Analog Output Voltage Test in"=refnum<class "Modulated Analog Output Voltage Test.lvclass"> refnum ("Constant Analog Input Voltage Test.lvclass"), "Test Values"=w278, "ConvertStrategy"=w271, "Tolerance"=w276, "Samples To Average"=w275, "error in (no error)"=w270, "DAQ Channel"=w279, "ConfigureILCStrategy"=refnum<class "ConfigureILCDAC1Strategy.lvclass"> refnum ("ConfigureILCDAC1Strategy.lvclass"), "Test Scenario"=TestScenarioTypes."DAC3 Test", "ILC"=w274, "Signal Name"="DAC3", "Log"=w266) -> ("Constant Analog Output Voltage Test  out"=w268:refnum<class "Modulated Analog Output Voltage Test.lvclass">, "error out"=w269:errorcluster)  [unwired: 6 in]
        }
        frame "DAC4 Test" {
          n65 = Unbundle By Name(w284) -> ("Analog Supply DAQ Channel to Read"=w283:refnum<k21>, "Samples To Average"=w291:i32)
          n66 = Unbundle By Name(w284) -> ("DAC4 DAQ Channel to Read"=w298:refnum<k21>, "Test Values"=w297:T5)
          n67 = Unbundle By Name(w284) -> ("Tolerance"=w295:dbl, "Samples To Average"=w294:i32)
          n68 = Unbundle By Name(w284) -> ("ILC"=w293:refnum<class "ILC.lvclass">)
          n69 = call "init.vi"("error in (no error)"=w286, "Samples To Average"=w291, "+5VA Channel"=w283, "ConvertDACRawToEngStrategy in"=refnum<class "ConvertDACRawToEngStrategy.lvclass"> refnum ("ConvertDACRawToEngStrategy.lvclass")) -> ("error out"=w289:errorcluster, "ConvertDACRawToEngStrategy out"=w290:refnum<class "ConvertDACRawToEngStrategy.lvclass">)  [unwired: 6 in]
          n70 = call "init.vi"("Constant Analog Output Voltage Test in"=refnum<class "Modulated Analog Output Voltage Test.lvclass"> refnum ("Constant Analog Input Voltage Test.lvclass"), "Test Values"=w297, "ConvertStrategy"=w290, "Tolerance"=w295, "Samples To Average"=w294, "error in (no error)"=w289, "DAQ Channel"=w298, "ConfigureILCStrategy"=refnum<class "ConfigureILCDAC1Strategy.lvclass"> refnum ("ConfigureILCDAC1Strategy.lvclass"), "Test Scenario"=TestScenarioTypes."DAC4 Test", "ILC"=w293, "Signal Name"="DAC4", "Log"=w285) -> ("Constant Analog Output Voltage Test  out"=w287:refnum<class "Modulated Analog Output Voltage Test.lvclass">, "error out"=w288:errorcluster)  [unwired: 6 in]
        }
        frame "BIAS Test" {
          n71 = Unbundle By Name(w302) -> ("DAQ Channel to Read"=w310:refnum<k21>, "Expected Value"=w311:dbl, "Tolerance"=w312:dbl, "Samples To Average"=w313:i32)
          n72 = call "init.vi"("Constant Analog Output Voltage Test in"=refnum<class "Constant Analog Output Voltage Test.lvclass"> refnum ("Constant Analog Input Voltage Test.lvclass"), "DAQ Channel"=w310, "Expected Value"=w311, "Tolerance"=w312, "Samples To Average"=w313, "error in (no error)"=w305, "MustPass?"=FALSE, "Log"=w306, "Test Scenario"=TestScenarioTypes."BIAS Test", "Signal Name"="BIAS") -> ("Constant Analog Output Voltage Test  out"=w303:refnum<class "Constant Analog Output Voltage Test.lvclass">, "error out"=w304:errorcluster)  [unwired: 8 in]
        }
        frame "EXC1 Test" {
          n73 = Unbundle By Name(w319) -> ("EXC1 DAQ Channel to Read"=w323:refnum<k21>, "Expected Value"=w324:dbl, "Tolerance"=w325:dbl, "Samples To Average"=w326:i32)
          n74 = call "init.vi"("Constant Analog Output Voltage Test in"=refnum<class "Constant Analog Output Voltage Test.lvclass"> refnum ("Constant Analog Input Voltage Test.lvclass"), "DAQ Channel"=w323, "Expected Value"=w324, "Tolerance"=w325, "Samples To Average"=w326, "error in (no error)"=w317, "MustPass?"=FALSE, "Log"=w318, "Test Scenario"=TestScenarioTypes."EXC1 Test", "Signal Name"="EXC1") -> ("Constant Analog Output Voltage Test  out"=w315:refnum<class "Constant Analog Output Voltage Test.lvclass">, "error out"=w316:errorcluster)  [unwired: 8 in]
        }
        frame "EXC2 Test" {
          n75 = Unbundle By Name(w330) -> ("EXC2 DAQ Channel to Read"=w336:refnum<k21>, "Expected Value"=w337:dbl, "Tolerance"=w338:dbl, "Samples To Average"=w339:i32)
          n76 = call "init.vi"("Constant Analog Output Voltage Test in"=refnum<class "Constant Analog Output Voltage Test.lvclass"> refnum ("Constant Analog Input Voltage Test.lvclass"), "DAQ Channel"=w336, "Expected Value"=w337, "Tolerance"=w338, "Samples To Average"=w339, "error in (no error)"=w332, "MustPass?"=FALSE, "Log"=w331, "Test Scenario"=TestScenarioTypes."EXC2 Test", "Signal Name"="EXC2") -> ("Constant Analog Output Voltage Test  out"=w329:refnum<class "Constant Analog Output Voltage Test.lvclass">, "error out"=w328:errorcluster)  [unwired: 8 in]
        }
        frame "EXC3 Test" {
          n77 = Unbundle By Name(w341) -> ("EXC3 DAQ Channel to Read"=w349:refnum<k21>, "Expected Value"=w350:dbl, "Tolerance"=w351:dbl, "Samples To Average"=w352:i32)
          n78 = call "init.vi"("Constant Analog Output Voltage Test in"=refnum<class "Constant Analog Output Voltage Test.lvclass"> refnum ("Constant Analog Input Voltage Test.lvclass"), "DAQ Channel"=w349, "Expected Value"=w350, "Tolerance"=w351, "Samples To Average"=w352, "error in (no error)"=w344, "MustPass?"=FALSE, "Log"=w345, "Test Scenario"=TestScenarioTypes."EXC3 Test", "Signal Name"="EXC3") -> ("Constant Analog Output Voltage Test  out"=w342:refnum<class "Constant Analog Output Voltage Test.lvclass">, "error out"=w343:errorcluster)  [unwired: 8 in]
        }
        frame "EXC4 Test" {
          n79 = Unbundle By Name(w354) -> ("EXC4 DAQ Channel to Read"=w362:refnum<k21>, "Expected Value"=w363:dbl, "Tolerance"=w364:dbl, "Samples To Average"=w365:i32)
          n80 = call "init.vi"("Constant Analog Output Voltage Test in"=refnum<class "Constant Analog Output Voltage Test.lvclass"> refnum ("Constant Analog Input Voltage Test.lvclass"), "DAQ Channel"=w362, "Expected Value"=w363, "Tolerance"=w364, "Samples To Average"=w365, "error in (no error)"=w357, "MustPass?"=FALSE, "Log"=w358, "Test Scenario"=TestScenarioTypes."EXC4 Test", "Signal Name"="EXC4") -> ("Constant Analog Output Voltage Test  out"=w355:refnum<class "Constant Analog Output Voltage Test.lvclass">, "error out"=w356:errorcluster)  [unwired: 8 in]
        }
      }
    }
    frame Error {
    }
  }
  "error out" <- w2
  "TestScenarioFactory out" <- w5
  "ITestScenario.lvclass" <- w4
